vi "start.vi"() -> ()   [LabVIEW 2015]
panel:
  in  "VI路径 2":path
  out "水平刻度条":u8(slide) scale=0.0..100.0
  in  "VI路径":path=path "C:/Users/Administrator/Desktop/跳远项目上位机/登录界面/系统主界面 .vi"
  in  "文件（使用对话框）":path=path "C:/Users/Administrator/Desktop/跳远项目上位机/登录界面/user.txt"
  in  "?":bool
  in  "账号":string
  in  "密码":string
  # "系统登录"
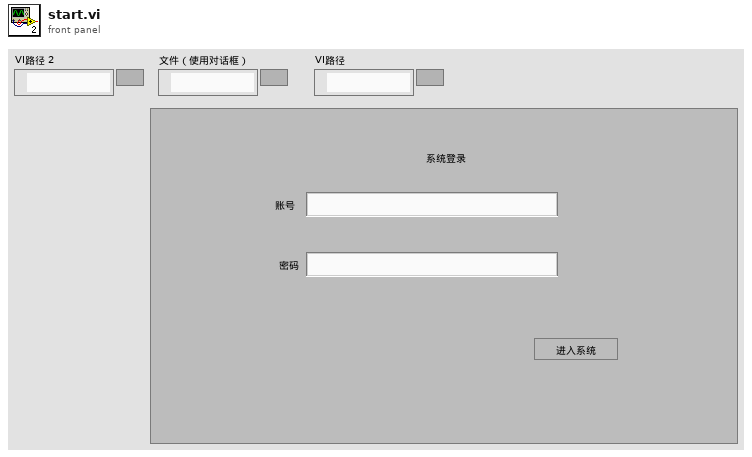
[diagram p1: front panel]
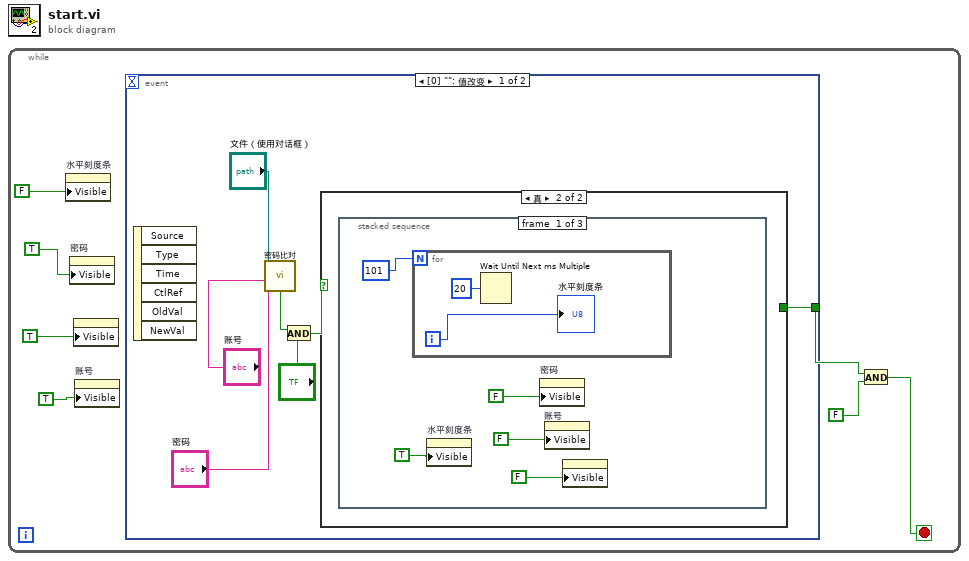
[diagram p0: block diagram]
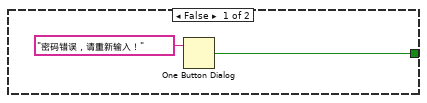
[diagram p2: hidden frame]
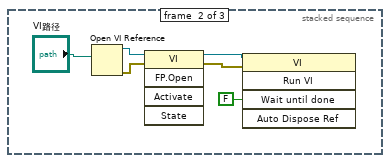
[diagram p3: hidden frame]
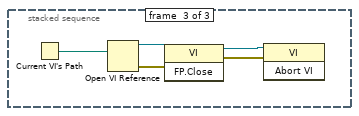
[diagram p4: hidden frame]
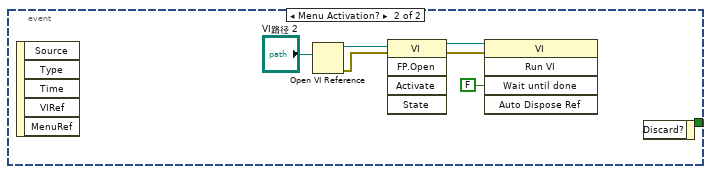
[diagram p5: hidden frame]
diagram:
  n1 = while {
    stop <- w5 stop-if-true
    n2 = property on="水平刻度条" class="Slide (严格)"("Visible"=FALSE ("可见")) -> ()  [unwired: 2 in, 2 out]
    n3 = property on="密码" class="Str"("Visible"=TRUE ("可见")) -> ()  [unwired: 2 in, 2 out]
    n4 = property class="Bool"("Visible"=TRUE ("可见")) -> ()  [unwired: 2 in, 2 out]
    n5 = property on="账号" class="Str"("Visible"=TRUE ("可见")) -> ()  [unwired: 2 in, 2 out]
    n6 = event shown="[0] \"\": 值改变" {
      selector: _ -> [_ _]
      dyn-events: _ -> [_ _]
      timeout: _ -> [_ _]
      tunnel: [w8 _] -> w7
      event Value Change {
        n7 = event-data() -> ()  [unwired: 1 in, 6 out]
        n8 = call "密码比对.vi"("密码"="密码", "账户"="账号", "文件（使用对话框）"="文件（使用对话框）") -> ("x = y?"=w11:bool)  [unwired: 8 in]
        n9 = And(x=w11, y="?") -> (x .and. y?=w9:bool)
        n10 = case shown="真" w9 {
          tunnel: [w15 _] -> w8
          frame False {
            n11 = One Button Dialog(message="密码错误，请重新输入！" ("消息")) -> (true=w15:bool)  [unwired: 1 in]
          }
          frame True {
            n12 = stacked-sequence {
              frame #0 {
                n13 = for {
                  N: 101 -> [_]
                  i -> [w23]
                  n14 = Wait Until Next ms Multiple(millisecond multiple=u32 20 ("毫秒倍数")) -> ()  [unwired: 1 out]
                  "水平刻度条" <- w23
                }
                n15 = property on="水平刻度条" class="Slide (严格)"("Visible"=TRUE ("可见")) -> ()  [unwired: 2 in, 2 out]
                n16 = property on="密码" class="Str"("Visible"=FALSE ("可见")) -> ()  [unwired: 2 in, 2 out]
                n17 = property on="账号" class="Str"("Visible"=FALSE ("可见")) -> ()  [unwired: 2 in, 2 out]
                n18 = property class="Bool"("Visible"=FALSE ("可见")) -> ()  [unwired: 2 in, 2 out]
              }
              frame #1 {
                n19 = Open VI Reference(vi path="VI路径") -> (vi reference=w27:refnum<vi>, error out=w28:errorcluster)  [unwired: 5 in]
                n20 = invoke class="VI" method="FP.Open"(reference=w27, error in=w28) -> (reference out=w26:refnum<vi>, error out=w25:errorcluster)  [unwired: 3 in, 3 out]
                n21 = invoke class="VI" method="Run VI"(reference=w26, error in=w25, "Wait until done"=FALSE ("结束前等待")) -> ()  [unwired: 2 in, 5 out]
              }
              frame #2 {
                n22 = Current VI's Path() -> (path=w34:path)
                n23 = Open VI Reference(vi path=w34) -> (vi reference=w32:refnum<vi>, error out=w33:errorcluster)  [unwired: 5 in]
                n24 = invoke class="VI" method="FP.Close"(reference=w32, error in=w33) -> (reference out=w31:refnum<vi>, error out=w30:errorcluster)  [unwired: 1 in, 1 out]
                n25 = invoke class="VI" method="Abort VI"(reference=w31, error in=w30) -> ()  [unwired: 1 in, 3 out]
              }
            }
          }
        }
      }
      event Menu Activation? {
        n26 = event-data() -> ()  [unwired: 1 in, 5 out]
        n27 = Open VI Reference(vi path="VI路径 2") -> (vi reference=w39:refnum<vi>, error out=w38:errorcluster)  [unwired: 5 in]
        n28 = invoke class="VI" method="FP.Open"(reference=w39, error in=w38) -> (reference out=w36:refnum<vi>, error out=w35:errorcluster)  [unwired: 3 in, 3 out]
        n29 = invoke class="VI" method="Run VI"(reference=w36, error in=w35, "Wait until done"=FALSE ("结束前等待")) -> ()  [unwired: 2 in, 5 out]
        n30 = event-data() -> ()  [unwired: 2 in, 1 out]
      }
    }
    n31 = And(x=w7, y=FALSE) -> (x .and. y?=w5:bool)
  }
